vi "电流测试TDK.vi"(0 "仪器实例 in":T1, 2 "电流测试点":dbl[](array[numeric]), 5 "error in (no error)":errorcluster) -> (13 "error out":errorcluster, 14 "仪器实例 out":T1, 15 "回读电流":dbl[](array[numeric]), 16 "输入电流":dbl[](array[numeric]), 17 "误差":dbl[](array[numeric]), 18 "斜率":dbl, 19 "截距":dbl)   [LabVIEW 2020]
uses:
  F:/F020/S7_1200 control/HslCommunication.dll
  S7_1200 control/HslCommunication.dll
  <vilib>/Analysis/NI_AALPro.lvlib
panel:
  out "数组 2":dbl[](array[numeric])
  out "数组":dbl[](array[numeric])
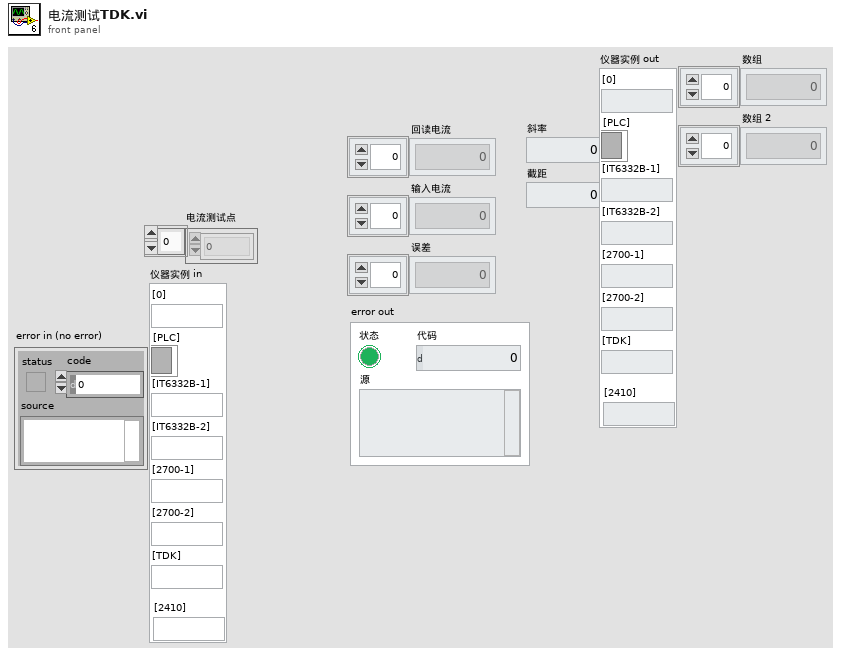
[diagram p1: front panel]
types:
  T1 = typedef "仪器实例.ctl" = cluster{"[0]":string, "[PLC]":refnum<k24>, "[IT6332B-1]":string, "[IT6332B-2]":string, "[2700-1]":string, "[2700-2]":string, "[TDK]":string, "[2410]":string}
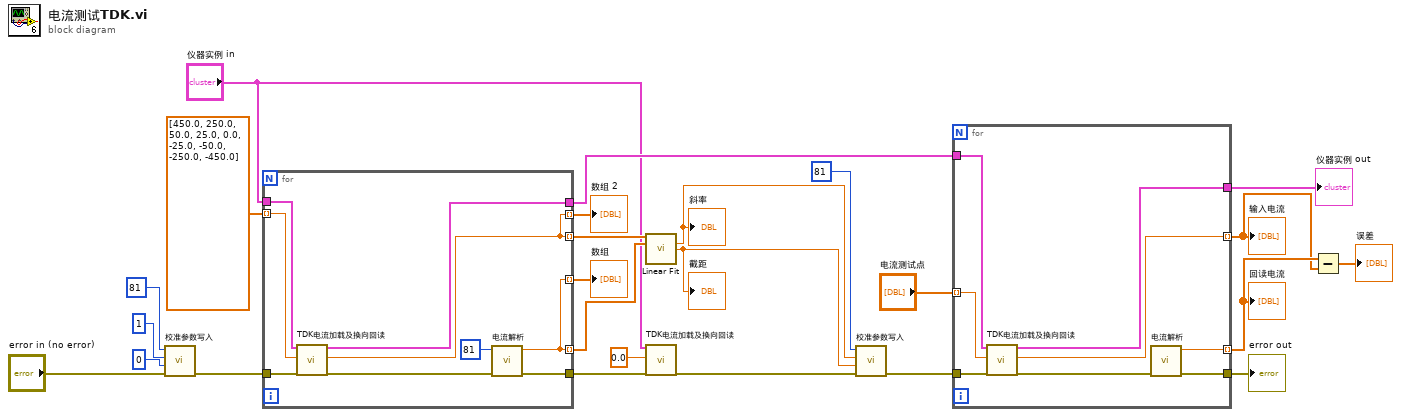
[diagram p0: block diagram]
diagram:
  n1 = call "校准参数写入.vi"("error in"="error in (no error)", "截距"=0, "斜率"=1, "Channel"=u16 81) -> ("error out"=w17:errorcluster)  [unwired: 6 in, 1 out]
  n2 = for {
    tunnel: dbl[] [450.0, 250.0, 50.0, 25.0, 0.0, -25.0, -50.0, -250.0, -450.0] ("Ramp Pattern") -> [w30] mode=indexing
    tunnel: w17 -> [w32]
    tunnel: [w27] -> w5 mode=indexing
    tunnel: [w33] -> w4
    tunnel: [w29] -> w23
    tunnel: "仪器实例 in" -> [w28]
    tunnel: [w27] -> w10 mode=indexing
    tunnel: [w26] -> w7 mode=indexing
    tunnel: [w26] -> w6 mode=indexing
    n3 = call "TDK电流加载及换向回读.vi"("仪器实例 in"=w28, "输入电流"=w30, "error in"=w32) -> ("仪器实例 out"=w29:T1, "实际电流"=w27:dbl, "error out"=w31:errorcluster)  [unwired: 14 in]
    n4 = call "电流解析.vi"("error in"=w31, "Channel"=u16 81) -> ("error out"=w33:errorcluster, "读取电流"=w26:dbl)  [unwired: 8 in]
  }
  "数组" <- w7
  "数组 2" <- w10
  n5 = call <vilib>:"Linear Fit.vi"("Y"=w5, "X"=w6) -> ("slope"=w8:dbl, "intercept"=w9:dbl)  [unwired: 9 in, 3 out]
  "斜率" <- w8
  "截距" <- w9
  n6 = call "TDK电流加载及换向回读.vi"("仪器实例 in"="仪器实例 in", "输入电流"=0.0, "error in"=w4) -> ("error out"=w1:errorcluster)  [unwired: 14 in, 2 out]
  n7 = call "校准参数写入.vi"("error in"=w1, "截距"=w9, "斜率"=w8, "Channel"=u16 81) -> ("error out"=w24:errorcluster)  [unwired: 6 in, 1 out]
  n8 = for {
    tunnel: "电流测试点" -> [w40] mode=indexing
    tunnel: w24 -> [w38]
    tunnel: w23 -> [w39]
    tunnel: [w42] -> w22 mode=indexing
    tunnel: [w36] -> w21 mode=indexing
    tunnel: [w41] -> w19
    tunnel: [w35] -> w12
    n9 = call "TDK电流加载及换向回读.vi"("仪器实例 in"=w39, "输入电流"=w40, "error in"=w38) -> ("仪器实例 out"=w35:T1, "实际电流"=w36:dbl, "error out"=w37:errorcluster)  [unwired: 14 in]
    n10 = call "电流解析.vi"("error in"=w37) -> ("error out"=w41:errorcluster, "读取电流"=w42:dbl)  [unwired: 9 in]
  }
  "回读电流" <- w22
  "输入电流" <- w21
  "error out" <- w19
  "仪器实例 out" <- w12
  n11 = Subtract(x=w22, y=w21) -> (x-y=→"误差":dbl[])
